vi "Get_Analog_Value_Two_Channels.vi"(7 "error in":errorcluster, 9 "Samples qty (1)":i32=1, 10 "Device IN":T1) -> (0 "error out":errorcluster, 1 "channel 2":waveform(i32), 2 "channel 1":waveform(i32), 3 "Device OUT":T1)   [LabVIEW 2017]
uses:
  device.ctl
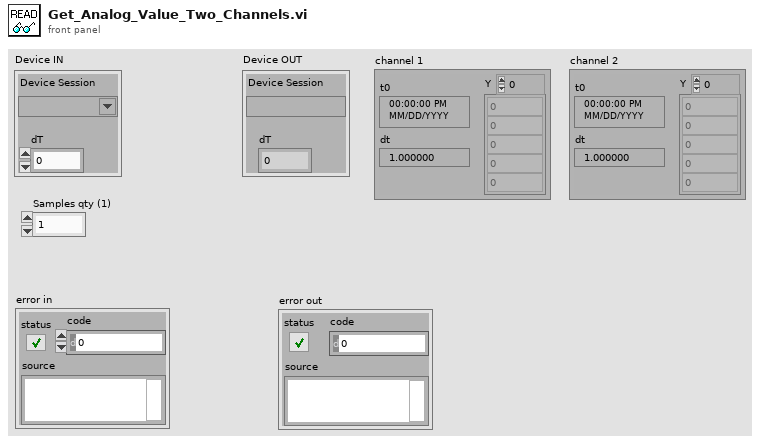
[diagram p1: front panel]
types:
  T1 = typedef "device.ctl" = cluster{"Device Session":refnum<visa-resource-name>, "dT":i32}
  T2 = cluster{"Device Session":refnum<visa-resource-name>, "dT":i32}
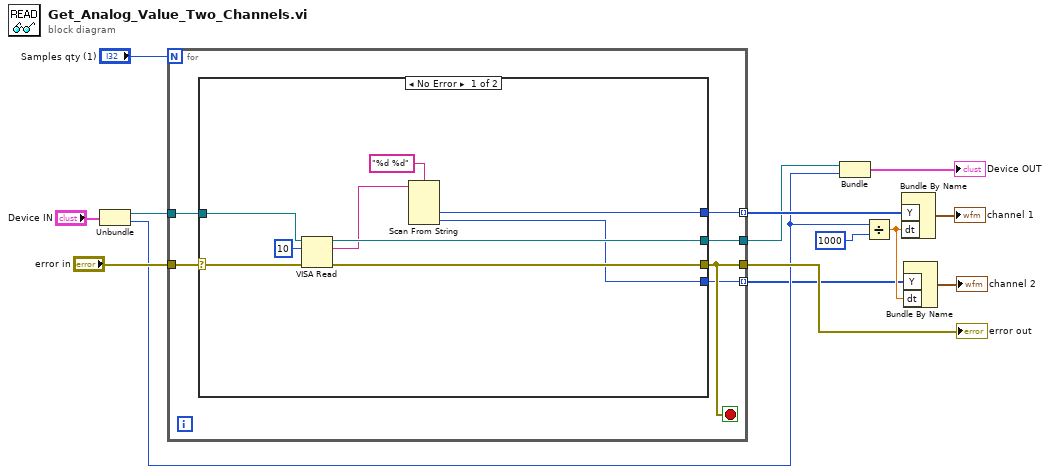
[diagram p0: block diagram]
diagram:
  n1 = Unbundle("Device IN") -> ("Device Session"=w8:refnum<visa-resource-name>, "dT"=w6:i32)
  n2 = for {
    N: "Samples qty (1)" -> [_]
    tunnel: [w20] -> w7
    tunnel: [w17] -> w14
    tunnel: [w19] -> w11 mode=indexing
    tunnel: "error in" -> [w18]
    tunnel: w8 -> [w16]
    tunnel: [w15] -> w1 mode=indexing
    stop <- w17 stop-if-true
    n3 = case shown="No Error" w18 {
      selector: w18 -> [w26 w31]
      tunnel: [w29 w31] -> w17
      tunnel: [w28 w30] -> w20
      tunnel: [w22 _] -> w19
      tunnel: w16 -> [w25 w30]
      tunnel: [w21 _] -> w15
      frame No Error {
        n4 = VISA Read(VISA resource name=w25, byte count=u32 10, error in (no error)=w26) -> (VISA resource name out=w28:refnum<visa-resource-name>, read buffer=w23:string, error out=w29:errorcluster)  [unwired: 1 out]
        n5 = Scan From String(format string="%d %d", input string=w23) -> (output 1=w22:i32, output 2=w21:i32)  [unwired: 4 in, 3 out]
      }
      frame Error {
      }
    }
  }
  "error out" <- w14
  n6 = Bundle("Device Session"=w7, "dT"=w6) -> (→"Device OUT":T2)  [unwired: 1 in]
  n7 = Divide(x=w6, y=u32 1000) -> (x/y=w2:dbl)
  n8 = Bundle By Name("Y"=w11, "dt"=w2) -> (→"channel 1":waveform(i32))  [unwired: 1 in]
  n9 = Bundle By Name("Y"=w1, "dt"=w2) -> (→"channel 2":waveform(i32))  [unwired: 1 in]
